vi "Obtain tabla estatus from Contabilidad.vi"(8 "error in (no error)":errorcluster, 10 "Tabla estatus":string[][](array[string]), 11 "UI in":refnum<class "UI.lvclass">) -> (0 "error out":errorcluster, 3 "UI out":refnum<class "UI.lvclass">)   [LabVIEW 2020, in "UI.lvlib" / "UI.lvclass"]
uses:
  UI.lvclass
  UI.lvclass/UI.ctl
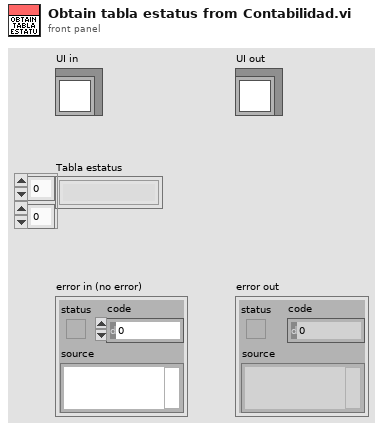
[diagram p1: front panel]
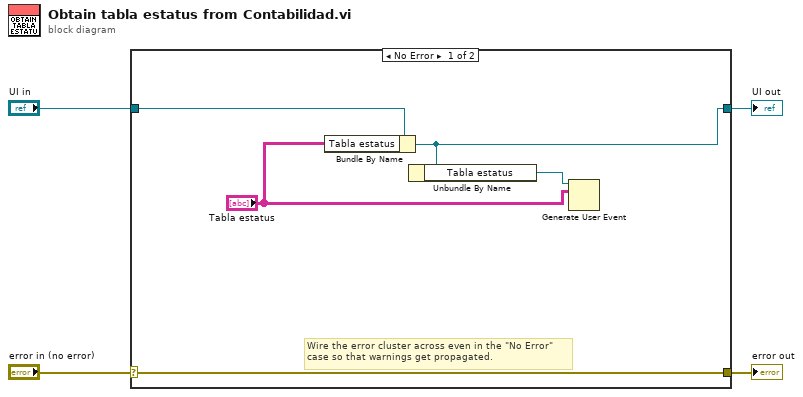
[diagram p0: block diagram]
diagram:
  n1 = case shown="No Error" "error in (no error)" {
    selector: "error in (no error)" -> [w9 w11]
    tunnel: [w9 w11] -> w3
    tunnel: [w7 w10] -> w1
    tunnel: "UI in" -> [w8 w10]
    frame No Error {
      # "Wire the error cluster across even in the \"No Error\"\ncase so that warnings get propagated."
      n2 = Bundle By Name(cluster=w8, "Tabla estatus"="Tabla estatus") -> (w7:refnum<class "UI.lvclass">)
      n3 = Unbundle By Name(w7) -> ("Tabla estatus"=w6:refnum<user-event>)
      n4 = Generate User Event(user event=w6, event data cluster="Tabla estatus") -> ()  [unwired: 2 in, 2 out]
    }
    frame Error {
    }
  }
  "error out" <- w3
  "UI out" <- w1
